vi "Check_G3.vi"(0 "trimmed string":string) -> (2 "G2 or G02":bool)   [LabVIEW 2017]
panel:
  out "output string 3":string
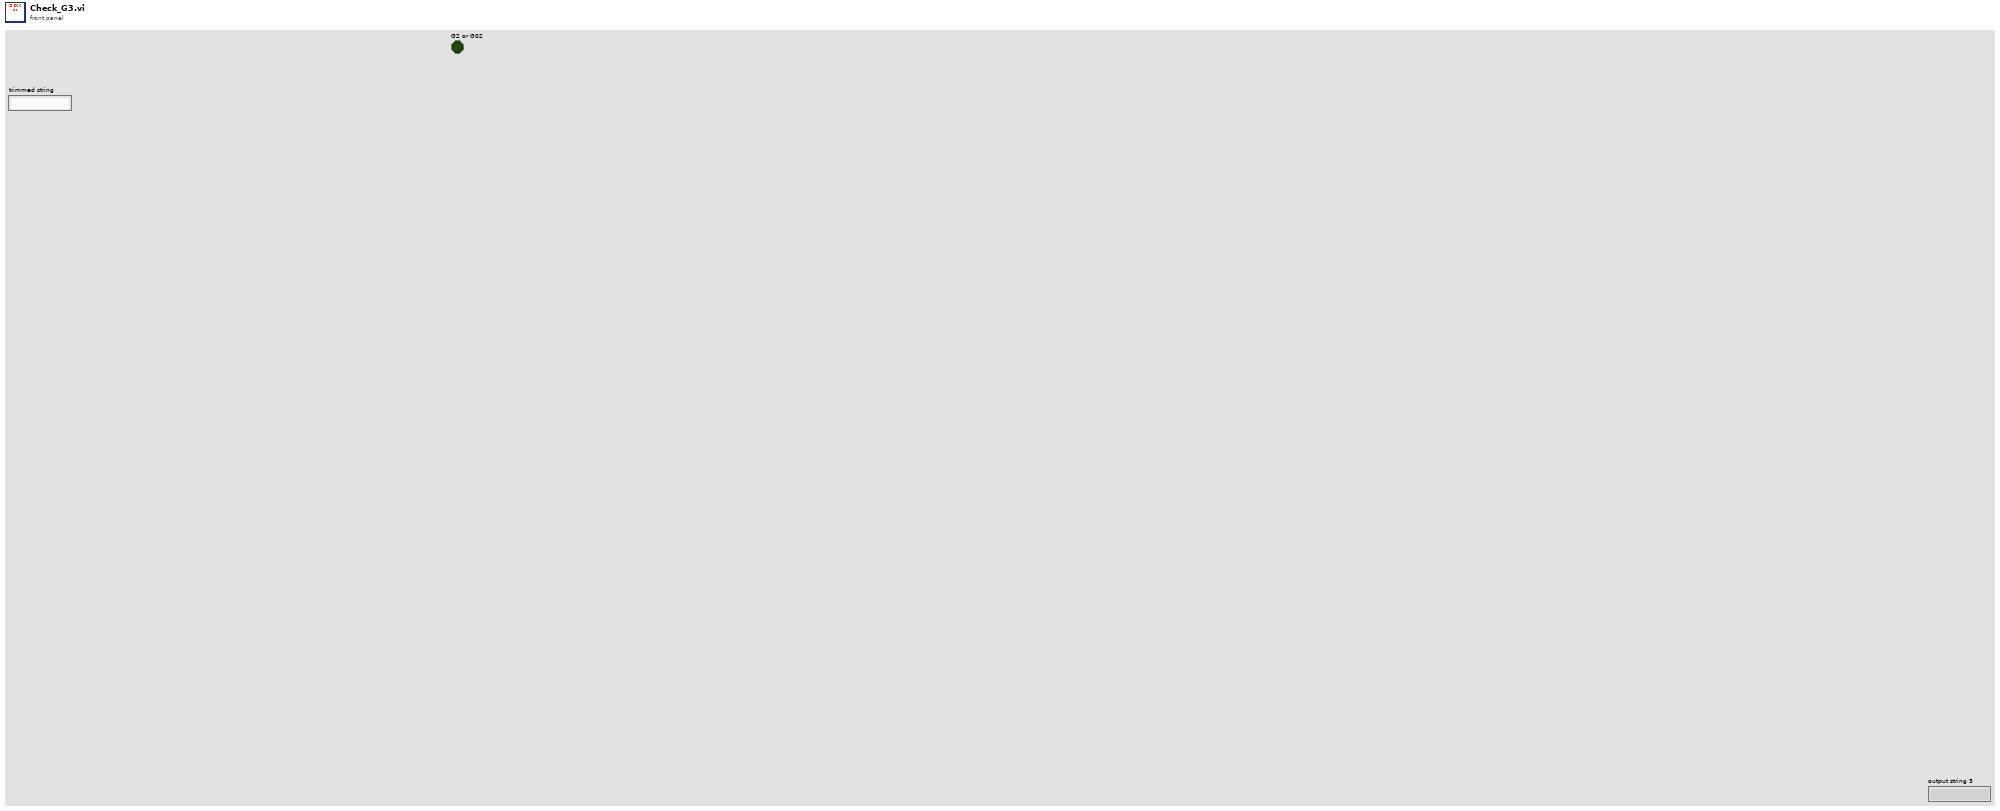
[diagram p1: front panel]
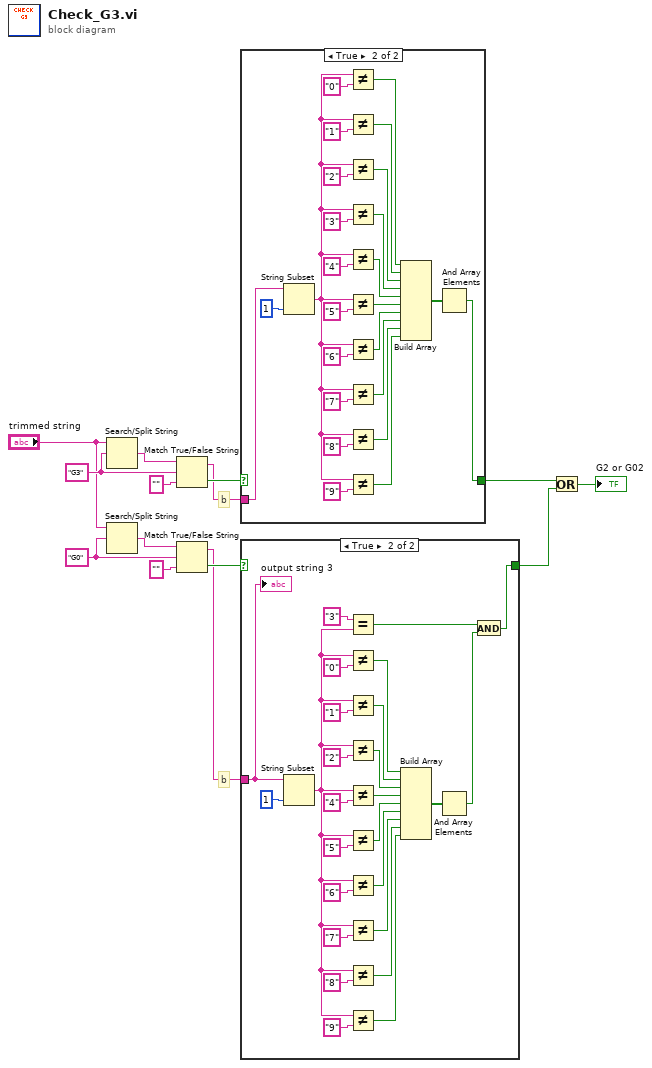
[diagram p0: block diagram]
diagram:
  w6 = "G0" ("true string")
  w11 = "G3" ("true string")
  # "b"
  # "b"
  n1 = Search/Split String(string="trimmed string", search string/char (-)=w11) -> (match + rest of string=w10:string)  [unwired: 1 in, 2 out]
  n2 = Search/Split String(string="trimmed string", search string/char (-)=w6) -> (match + rest of string=w5:string)  [unwired: 1 in, 2 out]
  n3 = Match True/False String(2:"" ("false string"), 3:w11, 4:w10) -> (0:w13:bool, 1:w12:string)
  n4 = Match True/False String(2:"" ("false string"), 3:w6, 4:w5) -> (0:w8:bool, 1:w7:string)
  n5 = case shown="True" w13 {
    selector: w13 -> [w15 _]
    tunnel: w12 -> [_ w39]
    tunnel: [w15 w16] -> w2
    frame False {
    }
    frame True {
      n6 = String Subset(string=w39, length (rest)=1 ("length (rest)")) -> (substring=w18:string)  [unwired: 1 in]
      n7 = Not Equal?(x=w18, y="0" ("false string")) -> (x != y?=w17:bool)
      n8 = Not Equal?(x=w18, y="1" ("false string")) -> (x != y?=w29:bool)
      n9 = Not Equal?(x=w18, y="2" ("false string")) -> (x != y?=w28:bool)
      n10 = Not Equal?(x=w18, y="3" ("false string")) -> (x != y?=w27:bool)
      n11 = Not Equal?(x=w18, y="4" ("false string")) -> (x != y?=w26:bool)
      n12 = Not Equal?(x=w18, y="5" ("false string")) -> (x != y?=w25:bool)
      n13 = Not Equal?(x=w18, y="6" ("false string")) -> (x != y?=w24:bool)
      n14 = Not Equal?(x=w18, y="7" ("false string")) -> (x != y?=w23:bool)
      n15 = Not Equal?(x=w18, y="8" ("false string")) -> (x != y?=w22:bool)
      n16 = Not Equal?(x=w18, y="9" ("false string")) -> (x != y?=w21:bool)
      n17 = Build Array(w17, w29, w28, w27, w26, w25, w24, w23, w22, w21) -> (w20:bool[])
      n18 = And Array Elements(Boolean array=w20) -> (logical AND=w16:bool)
    }
  }
  n19 = case shown="True" w8 {
    selector: w8 -> [w41 _]
    tunnel: w7 -> [_ w66]
    tunnel: [w41 w42] -> w3
    frame False {
    }
    frame True {
      n20 = String Subset(string=w66, length (rest)=1 ("length (rest)")) -> (substring=w55:string)  [unwired: 1 in]
      n21 = Equal?(x="3" ("false string"), y=w55) -> (x = y?=w44:bool)
      n22 = Not Equal?(x=w55, y="0" ("false string")) -> (x != y?=w54:bool)
      n23 = Not Equal?(x=w55, y="1" ("false string")) -> (x != y?=w53:bool)
      n24 = Not Equal?(x=w55, y="2" ("false string")) -> (x != y?=w52:bool)
      n25 = Not Equal?(x=w55, y="4" ("false string")) -> (x != y?=w51:bool)
      n26 = Not Equal?(x=w55, y="5" ("false string")) -> (x != y?=w50:bool)
      n27 = Not Equal?(x=w55, y="6" ("false string")) -> (x != y?=w49:bool)
      n28 = Not Equal?(x=w55, y="7" ("false string")) -> (x != y?=w48:bool)
      n29 = Not Equal?(x=w55, y="8" ("false string")) -> (x != y?=w47:bool)
      n30 = Not Equal?(x=w55, y="9" ("false string")) -> (x != y?=w46:bool)
      n31 = Build Array(w54, w53, w52, w51, w50, w49, w48, w47, w46) -> (w45:bool[])
      n32 = And Array Elements(Boolean array=w45) -> (logical AND=w43:bool)
      n33 = And(x=w44, y=w43) -> (x .and. y?=w42:bool)
      "output string 3" <- w66
    }
  }
  n34 = Or(x=w2, y=w3) -> (x .or. y?=→"G2 or G02":bool)
